vi "Chirp-Synthesize.vi"(0 "Duration (ms)":dbl, 1 "Cal":T1, 5 "Fmin (kHz)":dbl, 7 "Fmax (kHz)":dbl, 9 "Compensate":bool, 11 "error in (no error)":errorcluster, 12 "Sampling rate (Hz)":dbl, 13 "Npts":i32) -> (4 "Data.WF":dbl[](array[numeric]), 15 "error out":errorcluster)   [LabVIEW 2020]
uses:
  <vilib>/Analysis/4window.llb/Hanning Window (DBL).vi
  <vilib>/Analysis/4window.llb/AllCosWindow (DBL).vi
  Utility VIs/Math VIs/dB to Linear (1D).vi
  Utility VIs/Math VIs/interp1 (2D).vi
  <vilib>/Analysis/NI_AALPro.lvlib
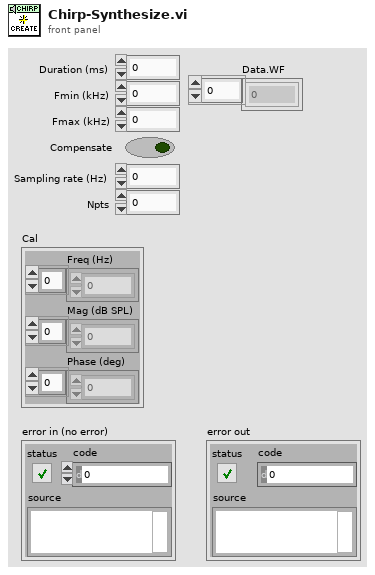
[diagram p1: front panel]
types:
  T1 = cluster{"Freq (Hz)":dbl[], "Mag (dB SPL)":dbl[], "Phase (deg)":dbl[]}
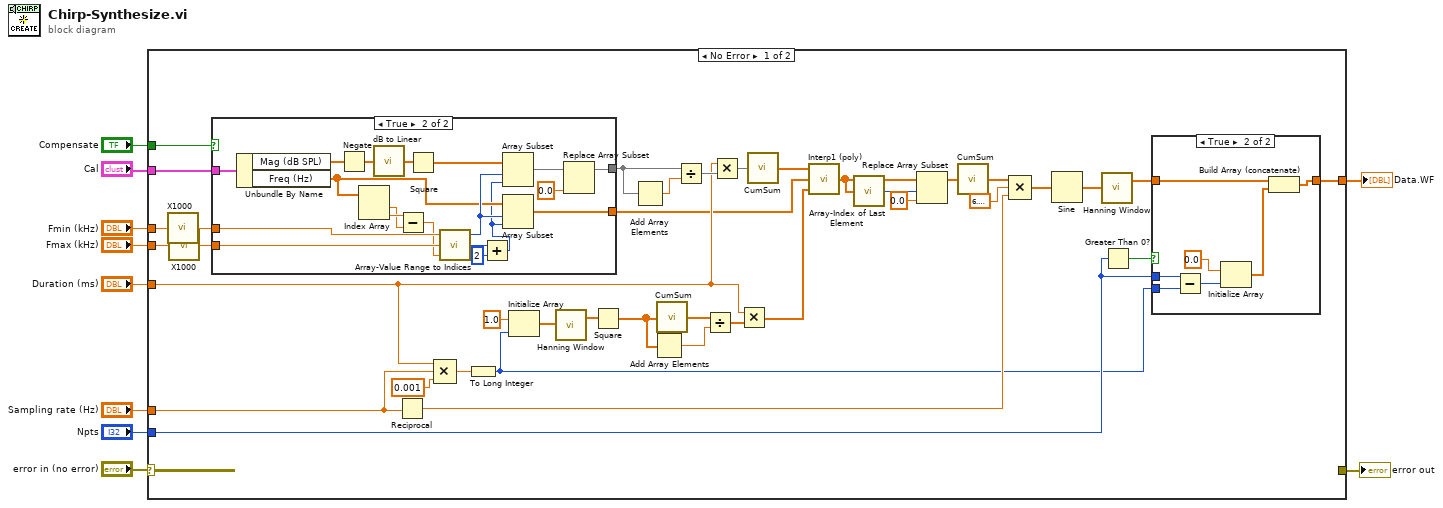
[diagram p0: block diagram]
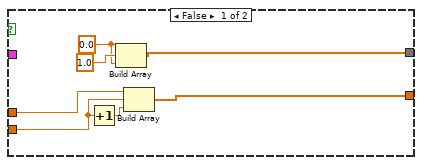
[diagram p3: hidden frame]
diagram:
  n1 = case shown="No Error" "error in (no error)" {
    selector: "error in (no error)" -> [_ w83]
    tunnel: [_ w83] -> w4
    tunnel: [w17 _] -> w5
    tunnel: "Duration (ms)" -> [w27 _]
    tunnel: "Fmin (kHz)" -> [w46 _]
    tunnel: "Fmax (kHz)" -> [w45 _]
    tunnel: "Compensate" -> [w48 _]
    tunnel: "Cal" -> [w47 _]
    tunnel: "Sampling rate (Hz)" -> [w34 _]
    tunnel: "Npts" -> [w19 _]
    frame No Error {
      n2 = call "X1000.vi"("X"=w46) -> ("X/1000"=w16:dbl)
      n3 = call "X1000.vi"("X"=w45) -> ("X/1000"=w15:dbl)
      n4 = case shown="True" w48 {
        tunnel: w47 -> [_ w82]
        tunnel: w16 -> [w63 w79]
        tunnel: w15 -> [w58 w78]
        tunnel: [w62 w74] -> w26
        tunnel: [w61 w67] -> w43
        frame False {
          w59 = 0.0
          n5 = Increment(x=w58) -> (x+1=w57:dbl)
          n6 = Build Array(w59, 1.0 ("element"), w59) -> (w61:dbl[])
          n7 = Build Array(w63, w58, w57) -> (w62:dbl[])
        }
        frame True {
          n8 = Unbundle By Name(w82) -> ("Mag (dB SPL)"=w73:dbl[], "Freq (Hz)"=w75:dbl[])
          n9 = Negate(x=w73) -> (-x=w71:dbl[])
          n10 = Index Array(array=w75) -> (element #1=w80:dbl, element #2=w81:dbl)  [unwired: 2 in]
          n11 = call-poly "dB to Linear.vi"("dB"=w71) -> ("linear"=w72:dbl[])
          n12 = Subtract(x=w81, y=w80) -> (x-y=w77:dbl)
          n13 = Square(x=w72) -> (x^2=w70:dbl[])
          n14 = call "Array-Value Range to Indices.vi"("dx"=w77, "Xmax"=w78, "Xmin"=w79) -> ("Length"=w66:i32, "Offset"=w76:i32)  [unwired: 1 in]
          n15 = Add(x=w66, y=2) -> (x+y=w65:i32)
          n16 = Array Subset(array=w70, index=w76, length=w65) -> (w68:dbl[])
          n17 = Array Subset(array=w75, index=w76, length=w65) -> (w74:dbl[])
          n18 = Replace Array Subset(array=w68, new element=0.0 ("new element/subarray")) -> (w67:dbl[])  [unwired: 1 in]
        }
      }
      n19 = Reciprocal(x=w34) -> (1/x=w33:dbl)
      n20 = Compound Arithmetic op=MULTIPLY(w27, w34, 0.001 ("value")) -> (w39:dbl)
      n21 = To Long Integer(number=w39) -> (32bit integer=w18:i32)
      n22 = Initialize Array(1.0 ("element"), w18) -> (w37:dbl[])
      n23 = call-poly <vilib>:"Hanning Window.vi"("X"=w37) -> ("Windowed X"=w22:dbl[])  [unwired: 1 out]
      n24 = Square(x=w22) -> (x^2=w36:dbl[])
      n25 = Add Array Elements(numeric array=w43) -> (sum=w44:dbl)
      n26 = Add Array Elements(numeric array=w36) -> (sum=w35:dbl)
      n27 = call "CumSum.vi"("Array"=w36) -> ("CumSum"=w28:dbl[])
      n28 = Divide(x=w43, y=w44) -> (x/y=w42:dbl[])
      n29 = Divide(x=w28, y=w35) -> (x/y=w24:dbl[])
      n30 = Multiply(x=w27, y=w42) -> (x*y=w41:dbl[])
      n31 = Multiply(x=w27, y=w24) -> (x*y=w23:dbl[])
      n32 = call "CumSum.vi"("Array"=w41) -> ("CumSum"=w25:dbl[])
      n33 = call-poly "Interp1 (poly).vi"("X"=w25, "Y"=w26, "U"=w23) -> ("V"=w12:dbl[])  [unwired: 2 in]
      n34 = call "Array-Index of Last Element.vi"("Array"=w12) -> ("Last Index"=w11:i32)
      n35 = Replace Array Subset(array=w12, new element=0.0 ("new element/subarray"), index=w11) -> (w14:dbl[])
      n36 = call "CumSum.vi"("Array"=w14) -> ("CumSum"=w29:dbl[])
      n37 = Compound Arithmetic op=MULTIPLY(w29, 6.283185307179586, w33) -> (w31:dbl[])
      n38 = Sine(x=w31) -> (sin(x)=w30:dbl[])
      n39 = call-poly <vilib>:"Hanning Window.vi"("X"=w30) -> ("Windowed X"=w21:dbl[])  [unwired: 1 out]
      n40 = Greater Than 0?(x=w19) -> (x > 0?=w20:bool)
      n41 = case shown="True" w20 {
        tunnel: w21 -> [w49 w52]
        tunnel: w19 -> [_ w56]
        tunnel: w18 -> [_ w55]
        tunnel: [w49 w50] -> w17
        frame False {
        }
        frame True {
          n42 = Subtract(x=w56, y=w55) -> (x-y=w54:i32)
          n43 = Initialize Array(0.0, w54) -> (w51:dbl[])
          n44 = Build Array (concatenate)(w52, w51) -> (w50:dbl[])
        }
      }
    }
    frame Error {
    }
  }
  "Data.WF" <- w5
  "error out" <- w4
